vi "NI VeriStand - Send Custom Device Message (Byte Array).vi"(6 "Timeout ms (5000)":i32=5000, 8 "error in (no error)":errorcluster, 9 "Data":u8[](array[numeric]), 10 "Command":string, 11 "Custom Device in":T1) -> (0 "error out":errorcluster, 1 "Response":u8[](array[numeric]), 3 "Custom Device out":T1)   [LabVIEW 2020, in "NI_VS Custom Device ExecutionAPI.lvlib"]
doc: "Sends a message or command to a custom device in an NI VeriStand project, as well as data required by the case that handles the command. You can use this VI with any custom device that registers to receive the <B>Command</B> you specify."
uses:
  <vilib>/NI VeriStand/Execution/CustomDevice/NI_VS Custom Device ExecutionAPI.lvlib
  <vilib>/NI VeriStand/Execution/CustomDevice/Custom Device Ref.ctl
  NationalInstruments.VeriStand.ClientAPI
  NationalInstruments.VeriStand
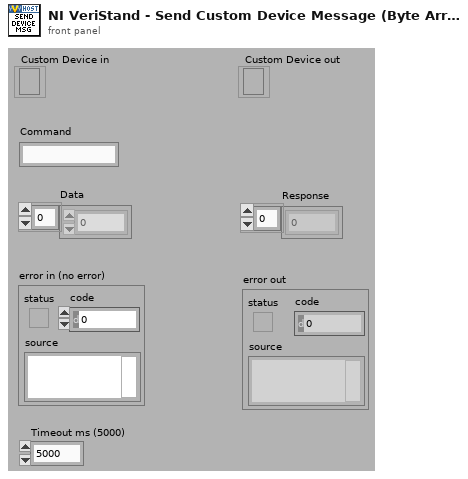
[diagram p1: front panel]
types:
  T1 = typedef "NI_VS Custom Device ExecutionAPI.lvlib/Custom Device Ref.ctl" = refnum<k24>
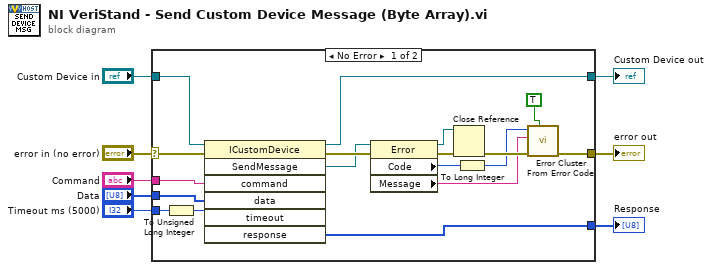
[diagram p0: block diagram]
diagram:
  n1 = case shown="No Error" "error in (no error)" {
    selector: "error in (no error)" -> [w24 w28]
    tunnel: [w13 w28] -> w8
    tunnel: "Custom Device in" -> [w12 w27]
    tunnel: [w11 w27] -> w5
    tunnel: "Timeout ms (5000)" -> [w17 _]
    tunnel: "Data" -> [w16 _]
    tunnel: "Command" -> [w15 _]
    tunnel: [w14 _] -> w1
    frame No Error {
      n2 = To Unsigned Long Integer(number=w17) -> (unsigned 32bit integer=w10:u32)
      n3 = invoke class="ICustomDevice" method="SendMessage"(reference=w12, error in=w24, "command"=w15, "data"=w16, "timeout"=w10) -> (reference out=w11:T1, error out=w25:errorcluster, "SendMessage"=w23:refnum<k24>, "response"=w14:u8[])  [unwired: 2 in, 3 out]
      n4 = property class="Error"(reference=w23, error in=w25) -> (reference out=w18:refnum<k24>, error out=w19:errorcluster, "Code"=w22:u32, "Message"=w21:string)
      n5 = Close Reference(reference=w18, error in (no error)=w19) -> (error out=w26:errorcluster)
      n6 = To Long Integer(number=w22) -> (32bit integer=w9:i32)
      n7 = call <vilib>:"Error Cluster From Error Code.vi"("show call chain? (False)"=TRUE, "error in (no error)"=w26, "error message (\"\")"=w21, "error code (0)"=w9) -> ("error out"=w13:errorcluster)  [unwired: 5 in]
    }
    frame Error {
    }
  }
  "Custom Device out" <- w5
  "error out" <- w8
  "Response" <- w1
